vi "DatastreamRead.vi"(8 "error in (no error)":errorcluster, 11 "connection ID":refnum<k16>) -> (0 "error out":errorcluster, 1 "Data Out":dbl[](array[numeric]), 3 "connection ID out":refnum<k16>)   [LabVIEW 2017]
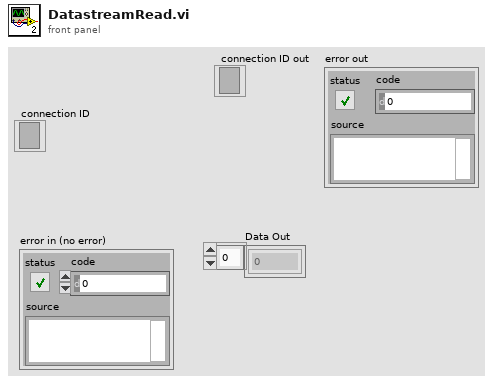
[diagram p1: front panel]
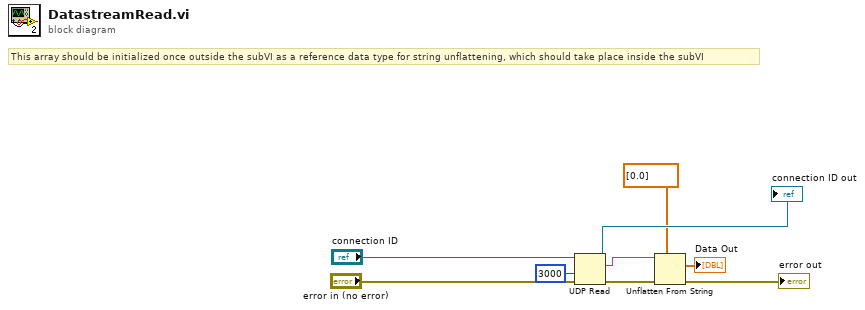
[diagram p0: block diagram]
diagram:
  # "This array should be initialized once outside the subVI as a reference data type for string unflattening, which should take place inside the subVI"
  n1 = UDP Read(connection ID="connection ID", timeout ms (25000)=3000, 8:"error in (no error)") -> (data out=w7:string, error out=w6:errorcluster, 3:→"connection ID out":refnum<k16>)  [unwired: 1 in, 2 out]
  n2 = Unflatten From String(type=dbl[] [0.0], binary string=w7, error in (no error)=w6) -> (value=→"Data Out":dbl[], error out=→"error out":errorcluster)  [unwired: 2 in, 1 out]
